vi "General triggers logic.vi"(8 "Trigger lines value":T4, 9 "PXI Trigger Enable":T1, 11 "Imaging Protocol":T2) -> (3 "Triggers output cluster":T3)   [LabVIEW 2020]
uses:
  <vilib>/eio/EIONode/EIONode.xnode
  <vilib>/rvi/eio/common/nirviEmuTemplateMethod_errors.vi
  FPGA Typedefs/Triggers output cluster.ctl
  FPGA Typedefs/PXI Trigger lines value cluster.ctl
  Typedefs/Imaging Protocols enum.ctl
  FPGA Typedefs/PXI Trigger Enable cluster.ctl
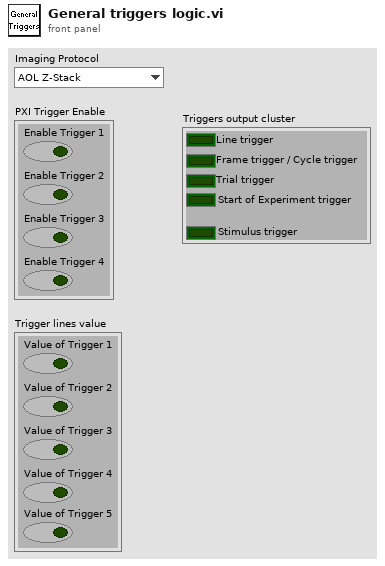
[diagram p1: front panel]
types:
  T1 = typedef "PXI Trigger Enable cluster.ctl" = cluster{"Enable Trigger 1":bool, "Enable Trigger 2":bool, "Enable Trigger 3":bool, "Enable Trigger 4":bool}
  T2 = typedef "Imaging Protocols enum.ctl" = enum16{"AOL Z-Stack", "Motor Z Stack", "Functional Acquisition", "Single Plane Acquisition", "Volume Acquisition", "Live Imaging", "Live Plane Imaging", "Live Volume Imaging"}
  T3 = typedef "Triggers output cluster.ctl" = cluster{"Line trigger":bool, "Frame trigger / Cycle trigger":bool, "Trial trigger":bool, "Start of Experiment trigger":bool, "Stimulus trigger":bool}
  T4 = typedef "PXI Trigger lines value cluster.ctl" = cluster{"Value of Trigger 1":bool, "Value of Trigger 2":bool, "Value of Trigger 3":bool, "Value of Trigger 4":bool, "Value of Trigger 5":bool}
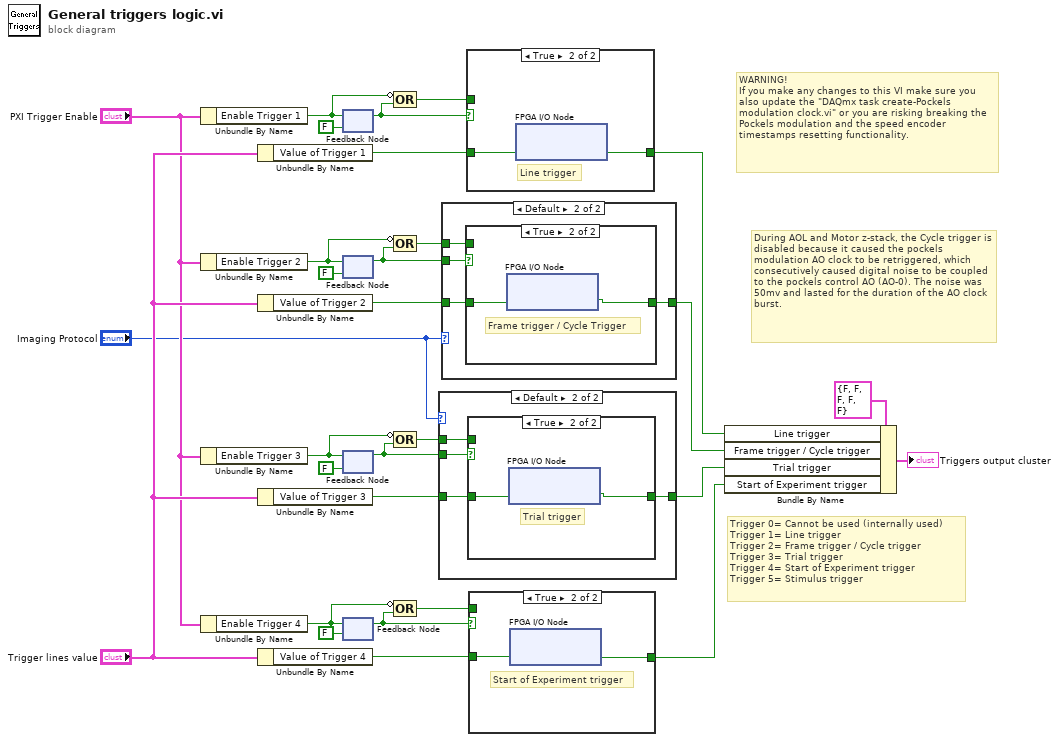
[diagram p0: block diagram]
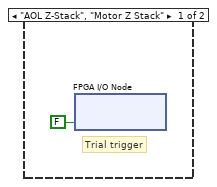
[diagram p2: hidden frame]
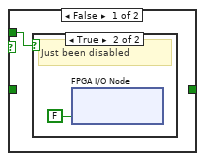
[diagram p3: hidden frame]
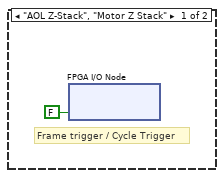
[diagram p5: hidden frame]
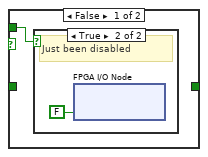
[diagram p6: hidden frame]
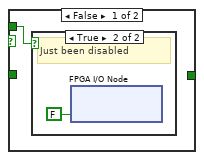
[diagram p8: hidden frame]
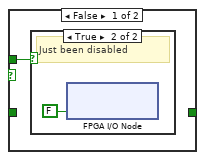
[diagram p10: hidden frame]
diagram:
  # "WARNING!\nIf you make any changes to this VI make sure you also update the \"DAQmx task create-Pockels modulation clock.vi\" or you are risking breaking the Pockels modulation and the speed encoder timestamps resetting functionality."
  # "Trigger 0= Cannot be used (internally used)\nTrigger 1= Line trigger\nTrigger 2= Frame trigger / Cycle trigger\nTrigger 3= Trial trigger\nTrigger 4= Start of Experiment trigger\nTrigger 5= Stimulus trigger"
  # "During AOL and Motor z-stack, the Cycle trigger is disabled because it caused the pockels modulation AO clock to be retriggered, which consecutively caused digital noise to be coupled to the pockels control AO (AO-0). The noise was 50mv and lasted for the duration of the AO clock burst."
  n1 = Unbundle By Name("PXI Trigger Enable") -> ("Enable Trigger 1"=w18:bool)
  n2 = Unbundle By Name("PXI Trigger Enable") -> ("Enable Trigger 2"=w21:bool)
  n3 = Unbundle By Name("PXI Trigger Enable") -> ("Enable Trigger 3"=w23:bool)
  n4 = Unbundle By Name("PXI Trigger Enable") -> ("Enable Trigger 4"=w25:bool)
  n5 = Unbundle By Name("Trigger lines value") -> ("Value of Trigger 1"=w6:bool)
  n6 = Unbundle By Name("Trigger lines value") -> ("Value of Trigger 2"=w5:bool)
  n7 = Unbundle By Name("Trigger lines value") -> ("Value of Trigger 3"=w4:bool)
  n8 = Unbundle By Name("Trigger lines value") -> ("Value of Trigger 4"=w3:bool)
  n9 = feedback #1(FALSE ("Trigger 1")) -> (w17:bool)
  n10 = feedback-in #1(w18) -> ()
  n11 = feedback #2(FALSE ("Trigger 2")) -> (w22:bool)
  n12 = feedback-in #2(w21) -> ()
  n13 = feedback #3(FALSE ("Trigger 3")) -> (w24:bool)
  n14 = feedback-in #3(w23) -> ()
  n15 = feedback #4(FALSE ("Trigger 4")) -> (w20:bool)
  n16 = feedback-in #4(w25) -> ()
  n17 = Compound Arithmetic op=OR(invert w18, w17) -> (w19:bool)
  n18 = Compound Arithmetic op=OR(invert w21, w22) -> (w26:bool)
  n19 = Compound Arithmetic op=OR(invert w23, w24) -> (w27:bool)
  n20 = Compound Arithmetic op=OR(invert w25, w20) -> (w28:bool)
  n21 = case shown="Default" "Imaging Protocol" {
    tunnel: w27 -> [_ w34]
    tunnel: w24 -> [_ w33]
    tunnel: [_ w32] -> w15
    tunnel: w4 -> [_ w31]
    frame "AOL Z-Stack", "Motor Z Stack" {
      # "Trial trigger"
      n22 = xnode "FPGA I/O Node"("PXI_Trig3"=FALSE ("PXI_Trig2")) -> ()  [unwired: 1 in, 1 out]
    }
    frame Default {
      n23 = case shown="True" w33 {
        tunnel: w31 -> [_ w37]
        tunnel: [_ w37] -> w32
        tunnel: w34 -> [w35 _]
        frame False {
          n24 = case shown="True" w35 {
            frame False {
              # "Idle"
            }
            frame True {
              # "Just been disabled"
              n25 = xnode "FPGA I/O Node"("PXI_Trig3"=FALSE ("PXI_Trig2")) -> ()  [unwired: 1 in, 1 out]
            }
          }
        }
        frame True {
          # "Trial trigger"
          n26 = xnode "FPGA I/O Node"("PXI_Trig3"=w37) -> ()  [unwired: 1 in, 1 out]
        }
      }
    }
  }
  n27 = case shown="Default" "Imaging Protocol" {
    tunnel: w5 -> [_ w42]
    tunnel: w22 -> [_ w41]
    tunnel: [_ w40] -> w14
    tunnel: w26 -> [_ w39]
    frame "AOL Z-Stack", "Motor Z Stack" {
      # "Frame trigger / Cycle Trigger"
      n28 = xnode "FPGA I/O Node"("PXI_Trig2"=FALSE) -> ()  [unwired: 1 in, 1 out]
    }
    frame Default {
      n29 = case shown="True" w41 {
        tunnel: w42 -> [_ w45]
        tunnel: [_ w45] -> w40
        tunnel: w39 -> [w43 _]
        frame False {
          n30 = case shown="True" w43 {
            frame False {
              # "Idle"
            }
            frame True {
              # "Just been disabled"
              n31 = xnode "FPGA I/O Node"("PXI_Trig2"=FALSE) -> ()  [unwired: 1 in, 1 out]
            }
          }
        }
        frame True {
          # "Frame trigger / Cycle Trigger"
          n32 = xnode "FPGA I/O Node"("PXI_Trig2"=w45) -> ()  [unwired: 1 in, 1 out]
        }
      }
    }
  }
  n33 = case shown="True" w17 {
    tunnel: w6 -> [_ w48]
    tunnel: [_ w48] -> w13
    tunnel: w19 -> [w46 _]
    frame False {
      n34 = case shown="True" w46 {
        frame False {
          # "Idle"
        }
        frame True {
          # "Just been disabled"
          n35 = xnode "FPGA I/O Node"("PXI_Trig1"=FALSE) -> ()  [unwired: 1 in, 1 out]
        }
      }
    }
    frame True {
      # "Line trigger"
      n36 = xnode "FPGA I/O Node"("PXI_Trig1"=w48) -> ()  [unwired: 1 in, 1 out]
    }
  }
  n37 = case shown="True" w20 {
    tunnel: w3 -> [_ w51]
    tunnel: [_ w51] -> w16
    tunnel: w28 -> [w49 _]
    frame False {
      n38 = case shown="True" w49 {
        frame False {
          # "Idle"
        }
        frame True {
          # "Just been disabled"
          n39 = xnode "FPGA I/O Node"("PXI_Trig4"=FALSE ("PXI_Trig2")) -> ()  [unwired: 1 in, 1 out]
        }
      }
    }
    frame True {
      # "Start of Experiment trigger"
      n40 = xnode "FPGA I/O Node"("PXI_Trig4"=w51) -> ()  [unwired: 1 in, 1 out]
    }
  }
  n41 = Bundle By Name(cluster=T3 {"Line trigger"=FALSE, "Frame trigger / Cycle trigger"=FALSE, "Trial trigger"=FALSE, "Start of Experiment trigger"=FALSE, "Stimulus trigger"=FALSE} ("Triggers output cluster"), "Line trigger"=w13, "Frame trigger / Cycle trigger"=w14, "Trial trigger"=w15, "Start of Experiment trigger"=w16) -> (→"Triggers output cluster":T3)
